vi "BYTE Size To DWORD Size.vi"(1 "BYTE Size":u32) -> (0 "DWORD Size":u32)   [LabVIEW 2014, in "Keyence LJ-V7000.lvlib"]
uses:
  Keyence LJ-V7000.lvlib
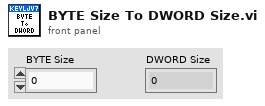
[diagram p1: front panel]
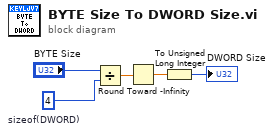
[diagram p0: block diagram]
diagram:
  w4 = u32 4  # sizeof(DWORD)
  n1 = Divide(x="BYTE Size", y=w4) -> (x/y=w3:dbl)
  n2 = Round Toward -Infinity(1:w3) -> (0:w2:dbl)
  n3 = To Unsigned Long Integer(number=w2) -> (unsigned 32bit integer=→"DWORD Size":u32)
